vi "LvMPDC_SUB_buildTreeView.vi"(8 "error in (no error)":errorcluster, 9 "Tag[]":cluster{"path":path, "Dir?":bool}[](array[cluster])=[{"path"=path "", "Dir?"=FALSE}, {"path"=path "", "Dir?"=FALSE}, {"path"=path "", "Dir?"=FALSE}, {"path"=path "", "Dir?"=FALSE}, {"path"=path "", "Dir?"=FALSE}, {"path"=path "", "Dir?"=FALSE}, {"path"=path "", "Dir?"=FALSE}], 11 "Tree Ref":refnum<vi>) -> (0 "error out":errorcluster, 3 "Tree Ref out":refnum<vi>)   [LabVIEW 2012]
panel:
  in  "path info":cluster{"path":path, "Dir?":bool}
  # "Tag配列のデータで、ツリー制御器を更新"
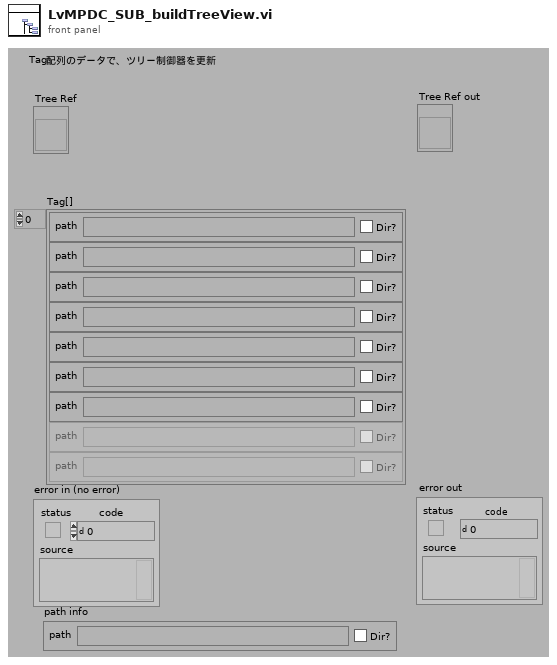
[diagram p1: front panel]
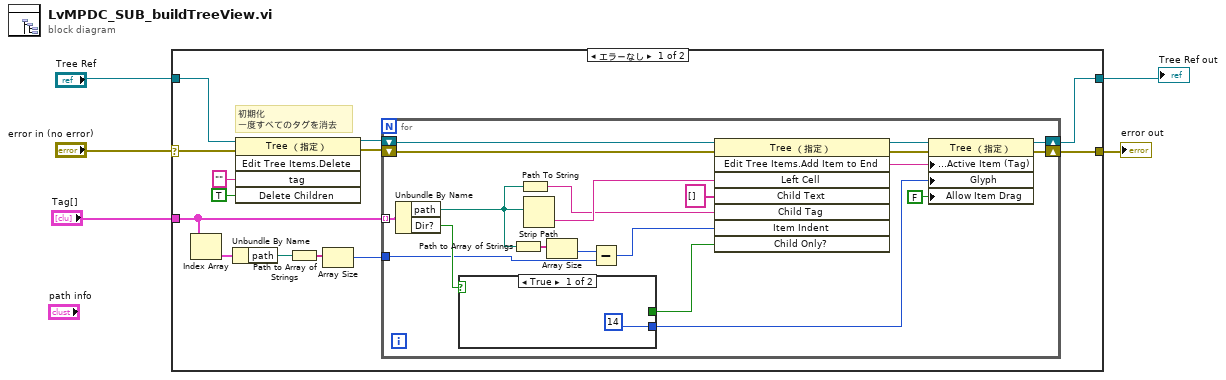
[diagram p0: block diagram]
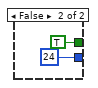
[diagram p2: hidden frame]
diagram:
  n1 = case shown="エラーなし" "error in (no error)" {
    selector: "error in (no error)" -> [w12 w42]
    tunnel: [w14 w43] -> w5
    tunnel: "Tree Ref" -> [w13 w43]
    tunnel: "Tag[]" -> [w10 _]
    tunnel: [w11 w42] -> w1
    frame No Error {
      # "初期化\n一度すべてのタグを消去"
      n2 = Index Array(array=w10) -> (element=w9:cluster{"path":path, "Dir?":bool})  [unwired: 1 in]
      n3 = Unbundle By Name(w9) -> ("path"=w7:path)
      n4 = invoke class="Tree （指定）" method="Edit Tree Items.Delete"(reference=w13, error in=w12, "tag"="" ("タグ"), "Delete Children"=TRUE ("子削除?")) -> (reference out=w16:refnum<vi>, error out=w15:errorcluster)  [unwired: 1 in, 3 out]
      n5 = Path to Array of Strings(0:w7) -> (2:w8:string[])  [unwired: 1 out]
      n6 = Array Size(array=w8) -> (size(s)=w6:i32)
      n7 = for {
        shift-right: [w34] -> w14
        shift-left: w16 -> [w38]
        shift-right: [w32] -> w11
        shift-left: w15 -> [w37]
        tunnel: w10 -> [w36] mode=indexing
        tunnel: w6 -> [w21]
        n8 = Unbundle By Name(w36) -> ("path"=w24:path, "Dir?"=w28:bool)
        n9 = case shown="TRUE" w28 {
          tunnel: [_ TRUE] -> w29
          tunnel: [14 ("アクティブ項目:記号指標") 24 ("アクティブ項目:記号指標")] -> w31
          frame True {
          }
          frame False {
          }
        }
        n10 = Path to Array of Strings(0:w24) -> (2:w23:string[])  [unwired: 1 out]
        n11 = Path To String(path=w24) -> (string=w25:string)
        n12 = Strip Path(path=w24) -> (name=w26:string)  [unwired: 1 out]
        n13 = Array Size(array=w23) -> (size(s)=w22:i32)
        n14 = Subtract(x=w22, y=w21) -> (x-y=w20:i32)
        n15 = invoke on="Invoke Node" class="Tree （指定）" method="Edit Tree Items.Add Item to End"(reference=w38, error in=w37, "Left Cell"=w26, "Child Text"=string[] [], "Child Tag"=w25, "Item Indent"=w20, "Child Only?"=w29) -> (reference out=w35:refnum<vi>, error out=w33:errorcluster, "Edit Tree Items:Add Item to End"=w19:string)  [unwired: 1 in, 5 out]
        n16 = property class="Tree （指定）"(reference=w35, error in=w33, "Active Item Properties:Active Item (Tag)"=w19, "Glyph"=w31, "Allow Item Drag"=FALSE) -> (reference out=w34:refnum<vi>, error out=w32:errorcluster)
      }
    }
    frame Error {
    }
  }
  "Tree Ref out" <- w5
  "error out" <- w1
